vi "Unregister by Name.vi"(7 "Event":refnum<class "Event.lvclass">, 8 "error in (no error)":errorcluster, 10 "Sink Name":string, 11 "Event Source in":refnum<class "Event Source.lvclass">) -> (0 "error out":errorcluster, 3 "Event Source out":refnum<class "Event Source.lvclass">)   [LabVIEW 2016, in "Event Source.lvlib" / "Event Source.lvclass"]
uses:
  Event Source.lvclass
  Event/Event.lvclass
  Event Source.lvclass/Event Source.ctl
  <vilib>/ActorFramework/Message Enqueuer/Message Enqueuer.lvclass
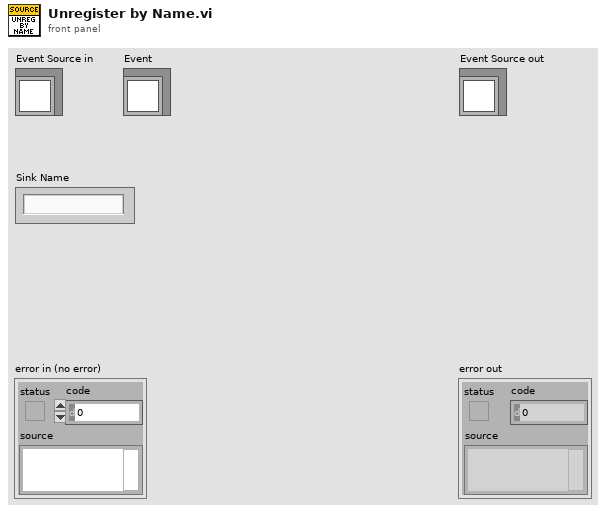
[diagram p1: front panel]
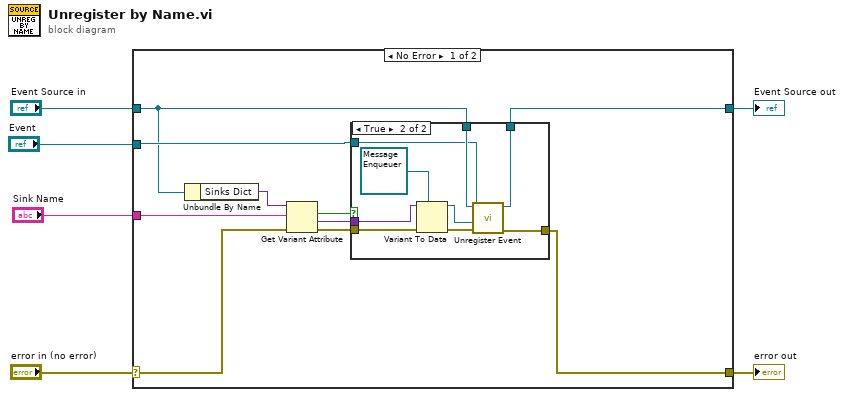
[diagram p0: block diagram]
diagram:
  n1 = case shown="No Error" "error in (no error)" {
    selector: "error in (no error)" -> [w8 w29]
    tunnel: [w7 w29] -> w5
    tunnel: [w9 w28] -> w3
    tunnel: "Event Source in" -> [w10 w28]
    tunnel: "Sink Name" -> [w15 _]
    tunnel: "Event" -> [w11 _]
    frame No Error {
      n2 = Unbundle By Name(w10) -> ("Sinks Dict"=w16:variant)
      n3 = Get Variant Attribute(Variant=w16, name=w15, error in=w8) -> (found=w14:bool, value=w13:variant, error out=w12:errorcluster)  [unwired: 1 in, 1 out]
      n4 = case shown="True" w14 {
        tunnel: w13 -> [_ w25]
        tunnel: w12 -> [w18 w26]
        tunnel: w10 -> [w17 w22]
        tunnel: w11 -> [_ w21]
        tunnel: [w18 w20] -> w7
        tunnel: [w17 w19] -> w9
        frame False {
        }
        frame True {
          n5 = Variant To Data(error in=w26, type=refnum<class "Message Enqueuer.lvclass"> refnum ("Actor's Enqueuer"), Variant=w25) -> (data=w23:refnum<class "Message Enqueuer.lvclass">, error out=w24:errorcluster)
          n6 = call "Unregister Event.vi"("Error In"=w24, "Registrant Address"=w23, "Event"=w21, "Event Source In"=w22) -> ("Error Out"=w20:errorcluster, "Event Source Out"=w19:refnum<class "Event Source.lvclass">)  [unwired: 6 in]
        }
      }
    }
    frame Error {
    }
  }
  "error out" <- w5
  "Event Source out" <- w3
